vi "Get Virt Instrs.vi"(8 "error in":errorcluster, 11 "MSS in":refnum<class "Measure and Stimulus Subsystems.lvclass">) -> (0 "error out":errorcluster, 2 "Virt Instr":T1(c390), 3 "MSS out":refnum<class "Measure and Stimulus Subsystems.lvclass">)   [LabVIEW 2023, in "HAL GOOP4.lvlib" / "Measure and Stimulus Subsystems.lvclass"]
uses:
  Measure and Stimulus Subsystems.lvclass
  Virt Instr Host/Virt Instr Local.lvclass
  Measure and Stimulus Subsystems.lvclass/Measure and Stimulus Subsystems.ctl
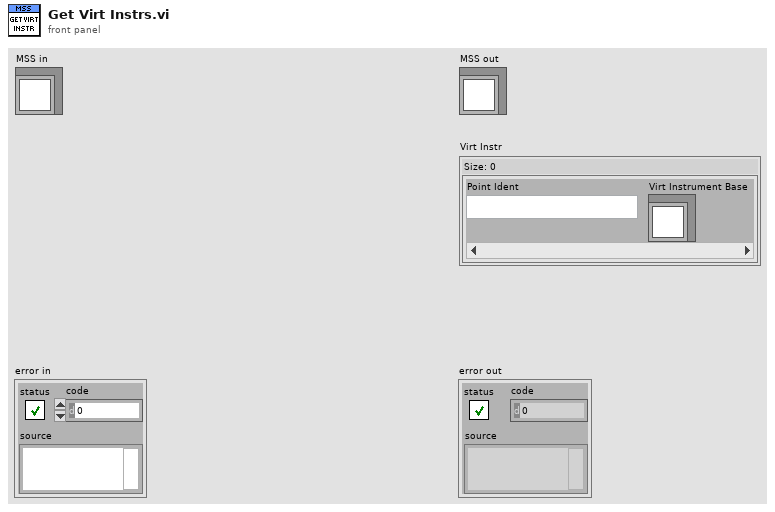
[diagram p1: front panel]
types:
  T1 = map{string, refnum<class "Virt Instr Local.lvclass">}
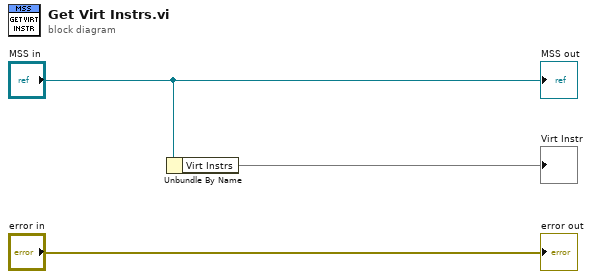
[diagram p0: block diagram]
diagram:
  n1 = Unbundle By Name("MSS in") -> ("Virt Instrs"=→"Virt Instr":T1)
  "error out" <- "error in"
  "MSS out" <- "MSS in"
